vi "_write_to_port.vi"(8 "error in (no error)":errorcluster, 10 "write buffer":string, 11 "Serial Port in":refnum<visa-resource-name>) -> (0 "error out":errorcluster, 3 "Serial Port out":refnum<visa-resource-name>)   [LabVIEW 2016, in "Chemyx_Syringe_Pump_driver.lvlib"]
doc: "Write the buffer to serial port in after adding end of line characters. Serial port out is a duplicate of Serial port in."
uses:
  Chemyx_Syringe_Pump_driver.lvlib
  <vilib>/Utility/error.llb/whitespace.ctl
panel:
  # "Write the buffer to serial port in after adding end of line characters. Serial port out is a duplicate of Serial port in."
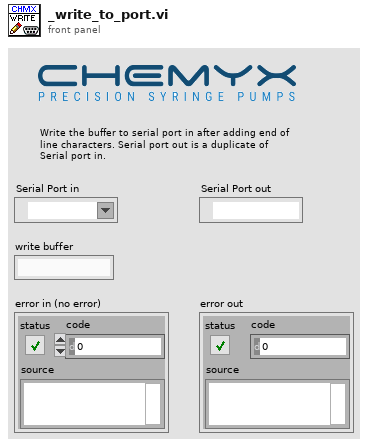
[diagram p1: front panel]
types:
  T1 = typedef "whitespace.ctl" = u16
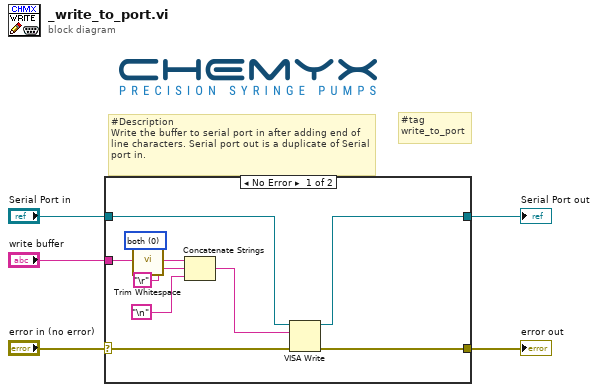
[diagram p0: block diagram]
diagram:
  # "#tag\nwrite_to_port"
  # "#Description\nWrite the buffer to serial port in after adding end of line characters. Serial port out is a duplicate of Serial port in."
  n1 = case shown="No Error" "error in (no error)" {
    selector: "error in (no error)" -> [w12 w17]
    tunnel: "write buffer" -> [w8 _]
    tunnel: [w14 w16] -> w4
    tunnel: [w13 w17] -> w3
    tunnel: "Serial Port in" -> [w11 w16]
    frame No Error {
      w6 = T1 0 items=["both", "start of string", "end of string"] ("location (both)")
      n2 = call <vilib>:"Trim Whitespace.vi"("string"=w8, "location (both)"=w6) -> ("trimmed string"=w7:string)
      n3 = Concatenate Strings(w7, "\r", "\n") -> (w9:string)
      n4 = VISA Write(VISA resource name=w11, write buffer=w9, error in (no error)=w12) -> (VISA resource name out=w14:refnum<visa-resource-name>, error out=w13:errorcluster)  [unwired: 1 out]
    }
    frame Error {
    }
  }
  "Serial Port out" <- w4
  "error out" <- w3
